vi "writeReadReg.vi"(6 "Bytes To Read":u8, 7 "I2C Channel":u8, 8 "error in":errorcluster, 9 "Data":u8[](array[numeric])=[0], 10 "I2C Slave Address":u8, 11 "LINX Resource in":T1) -> (0 "error out":errorcluster, 2 "Bytes Read":u8[](array[numeric]), 3 "LINX Resource out":T1)   [LabVIEW 2017]
uses:
  <vilib>/MakerHub/LINX/Private/Type Defs/LINX Ref.ctl
  <vilib>/MakerHub/LINX/Private/Type Defs/Platform.ctl
  <vilib>/MakerHub/LINX/Private/Type Defs/Interface.ctl
  <vilib>/MakerHub/LINX/Private/Device/Type Defs/LINX Device Config.ctl
  <vilib>/MakerHub/LINX/Private/Device/Type Defs/TCP Config.ctl
  <vilib>/MakerHub/LINX/Private/Device/Type Defs/Channels.ctl
  <vilib>/myRIO/Instrument Drivers/Onboard IO/I2C/typedefs/I2C User Configuration.ctl
  <vilib>/myRIO/Instrument Drivers/Onboard IO/I2C/typedefs/I2C Transfer Rate.ctl
  <vilib>/myRIO/Instrument Drivers/Onboard IO/I2C/typedefs/I2C Reference.ctl
  <vilib>/myRIO/Common/Instrument Driver Framework/Utilities/typedefs/myRIO Generic Hardware Reference.ctl
  <vilib>/myRIO/Common/Instrument Driver Framework/Utilities/typedefs/Hardware Version Enum.ctl
  <vilib>/myRIO/Common/Instrument Driver Framework/Utilities/typedefs/myRIO v1.0 Reference.ctl
  <vilib>/myRIO/Common/Instrument Driver Framework/Utilities/typedefs/Generic FPGA Reference.ctl
  <vilib>/myRIO/Common/Instrument Driver Framework/myRIO v1.0/I2C/typedefs/I2C Channels Enum.ctl
  <vilib>/myRIO/Instrument Drivers/Onboard IO/I2C/typedefs/I2C Configuration.ctl
  <vilib>/userdefined/High Color/nirio_resource_hc.ctl
  <vilib>/myRIO/Common/Instrument Driver Framework/Utilities/vis/Is FPGA Ref Available.vi
  <vilib>/myRIO/Common/Instrument Driver Framework/myRIO v1.0/I2C/vis/myRIO v1.1 Open I2C.vi
  <vilib>/MakerHub/LINX/Private/Local IO/LinxI2cWrite.vi
  <vilib>/MakerHub/LINX/Public/Utilities/Check Channel.vi
  <vilib>/myRIO/Common/Instrument Driver Framework/Utilities/vis/Validate Channels.vi
  <vilib>/myRIO/Common/Instrument Driver Framework/myRIO v1.0/I2C/vis/myRIO v1.0 Reserve I2C.vi
  <vilib>/myRIO/Common/Instrument Driver Framework/myRIO v1.0/I2C/vis/myRIO v1.0 Build MUX Configuration I2C.vi
  <vilib>/myRIO/Common/Instrument Driver Framework/myRIO v1.0/Resource Manager/vis/myRIO v1.0 Reserve Channel List.vi
  <vilib>/myRIO/Common/Instrument Driver Framework/myRIO v1.0/Resource Manager/vis/myRIO v1.0 Create Configuration List.vi
  <vilib>/myRIO/Common/Instrument Driver Framework/myRIO v1.0/Resource Manager/vis/myRIO v1.0 Reserve Channel.vi
  <vilib>/myRIO/Common/Instrument Driver Framework/myRIO v1.0/Resource Manager/vis/myRIO v1.0 Unreserve Channel.vi
  <vilib>/myRIO/Common/Instrument Driver Framework/myRIO v1.0/Resource Manager/vis/myRIO v1.0 Build Mutex Name.vi
  <vilib>/MakerHub/LINX/Private/Utilties/Generate Error.vi
  <vilib>/Utility/VariantDataType/GetNumericInfo.vi
  <vilib>/Utility/error.llb/Error Cluster From Error Code.vi
  <vilib>/myRIO/Common/Instrument Driver Framework/myRIO v1.0/myRIO v1.1 Open.vi
  <vilib>/myRIO/Common/Instrument Driver Framework/Utilities/vis/IO Manager.vi
  <vilib>/myRIO/Common/Instrument Driver Framework/Utilities/vis/Configuration Manager.vi
  <vilib>/myRIO/Common/Instrument Driver Framework/myRIO v1.0/Resource Manager/vis/myRIO v1.0 Configure IO.vi
  <vilib>/myRIO/Common/Instrument Driver Framework/myRIO v1.0/myRIO v1.0 Close.vi
  <vilib>/myRIO/Common/Instrument Driver Framework/myRIO v1.0/I2C/vis/myRIO v1.0 Configure I2C.vi
  <vilib>/myRIO/Common/Instrument Driver Framework/myRIO v1.0/I2C/vis/myRIO v1.0 Write I2C.vi
  <vilib>/myRIO/Common/Instrument Driver Framework/myRIO v1.0/I2C/vis/myRIO v1.0 Read I2C.vi
  <vilib>/myRIO/Express VI/Onboard IO/I2C/I2C Express VI.xnode
  <vilib>/myRIO/Instrument Drivers/Onboard IO/I2C/vis/myRIO I2C Open.xnode
  <vilib>/myRIO/Instrument Drivers/Onboard IO/I2C/I2C.lvlib
  <vilib>/MakerHub/LINX/LMH-LINX.lvlib
  <vilib>/MakerHub/LINX/Private/Device/Device.lvlib
panel:
  in  "I2C Impl.":enum16{"LINX", "myRIO Express", "myRIO subVIs"}(ring)=enum."myRIO subVIs"
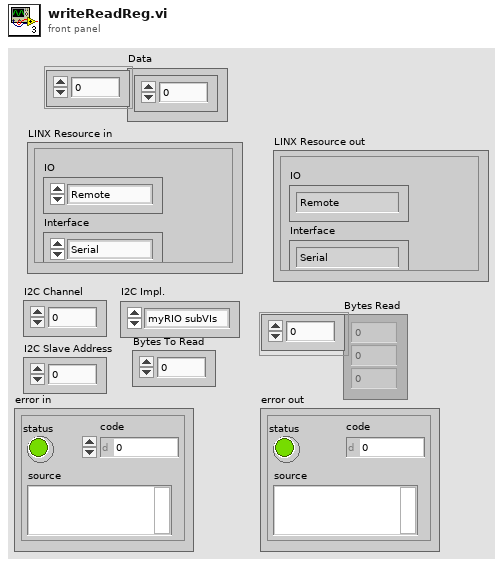
[diagram p1: front panel]
types:
  T1 = typedef "LMH-LINX.lvlib/LINX Ref.ctl" = cluster{"IO":T2, "Interface":T3, "LINX Device Config":T4}
  T2 = typedef "LMH-LINX.lvlib/Platform.ctl" = enum16{"Remote", "Local"}
  T3 = typedef "LMH-LINX.lvlib/Interface.ctl" = enum16{"Serial", "TCP"}
  T4 = typedef "LMH-LINX.lvlib/Device.lvlib/LINX Device Config.ctl" = cluster{"Interface":T3, "COM Port":refnum<visa-resource-name>, "TCP Configuration":T5, "Device Family":u8, "Device ID":u8, "Device Name":string, "TCP Ref":refnum<k5>, "Channels":T6}
  T5 = typedef "LMH-LINX.lvlib/Device.lvlib/TCP Config.ctl" = cluster{"IP Address":string, "Port":u16}
  T6 = typedef "LMH-LINX.lvlib/Channels.ctl" = cluster{"DI":u8[], "DO":u8[], "AI":u8[], "AO":u8[], "PWM":u8[], "QE":u8[], "UART":u8[], "I2C 2":u8[], "SPI":u8[], "CAN":u8[], "Servo":u8[], "AI Ref (V)":dbl, "AI Resolution (Bits)":u8, "AO Ref (V)":dbl, "AO Resolution (Bits)":u8}
  T7 = typedef "I2C.lvlib/I2C Reference.ctl" = cluster{"myRIO Reference":T8, "I2C Channels Enum":T12, "I2C Configuration":T13}
  T8 = typedef "myRIO Generic Hardware Reference.ctl" = cluster{"myRIO Model":T9, "myRIO Hardware Reference":T10}
  T9 = typedef "Hardware Version Enum.ctl" = enum16{"Unknown", "myRIO-1900", "myRIO-1950", "roboRIO", "NI ELVIS RIO CM"}
  T10 = typedef "myRIO v1.0 Reference.ctl" = cluster{"Generic FPGA Reference":T11, "Allow multiple opens":bool}
  T11 = typedef "Generic FPGA Reference.ctl" = refnum<k20>
  T12 = typedef "I2C Channels Enum.ctl" = enum16{"Not Connected", "A/I2C", "B/I2C", "I2C/I2C"}
  T13 = typedef "I2C.lvlib/I2C Configuration.ctl" = cluster{"I2C Transfer Rate":T14}
  T14 = typedef "I2C.lvlib/I2C Transfer Rate.ctl" = enum16{"Standard mode (100 kbps)", "Fast mode (400 kbps)"}
  T15 = typedef "I2C.lvlib/I2C User Configuration.ctl" = cluster{"I2C Transfer Rate":T14}
  T16 = typedef "nirio_resource_hc.ctl" = tag
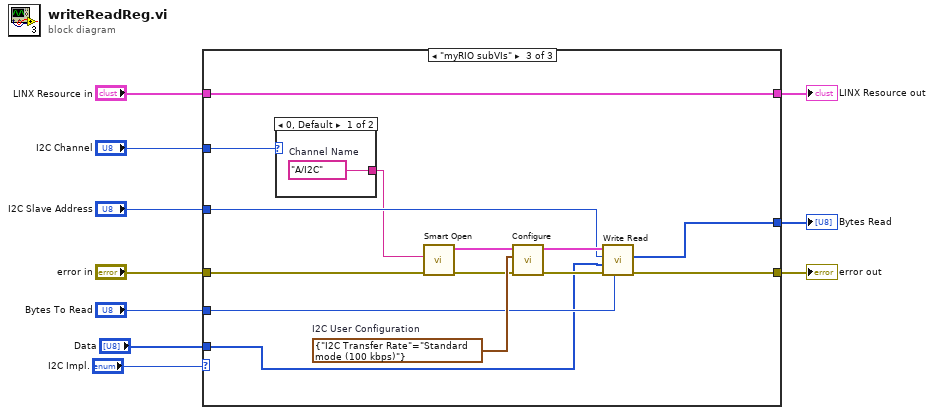
[diagram p0: block diagram]
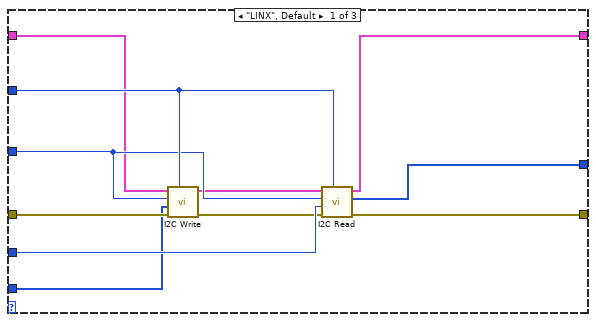
[diagram p2: hidden frame]
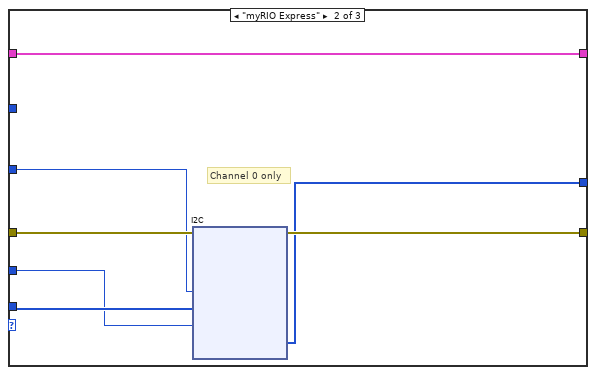
[diagram p3: hidden frame]
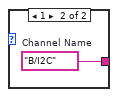
[diagram p4: hidden frame]
diagram:
  n1 = case shown="\"myRIO subVIs\"" "I2C Impl." {
    tunnel: [w20 w25 w81] -> w10
    tunnel: "error in" -> [w16 w27 w76]
    tunnel: [w21 w26 w69] -> w8
    tunnel: "I2C Slave Address" -> [w13 w24 w75]
    tunnel: "Bytes To Read" -> [w18 w22 w74]
    tunnel: "I2C Channel" -> [w14 _ w73]
    tunnel: "LINX Resource in" -> [w12 w28 w72]
    tunnel: [w19 w28 w72] -> w2
    tunnel: "Data" -> [w15 w23 w71]
    frame "LINX", Default {
      n2 = call <vilib>:"I2C Write.vi"("I2C Channel"=w14, "Error In"=w16, "Data"=w15, "I2C Slave Address (0)"=w13, "LINX Resource"=w12) -> ("Error Out"=w17:errorcluster, "LINX Resource"=w11:T1)  [unwired: 5 in]
      n3 = call <vilib>:"I2C Read.vi"("I2C Channel"=w14, "Error In"=w17, "Bytes To Read"=w18, "I2C Slave Address (0)"=w13, "LINX Resource"=w11) -> ("Error Out"=w21:errorcluster, "Data"=w20:u8[], "LINX Resource"=w19:T1)  [unwired: 4 in]
    }
    frame "myRIO Express" {
      # "Channel 0 only"
      n4 = xnode "I2C"("Slave Address (7-bit)"=w24, "Bytes to Write"=w23, "Byte Count"=w22, "error in (no error)"=w27) -> ("Bytes Read"=w25:u8[], "error out"=w26:errorcluster)
    }
    frame "myRIO subVIs" {
      w82 = T15 {"I2C Transfer Rate"=enum."Standard mode (100 kbps)"}  # I2C User Configuration
      n5 = case shown="0, Default" w73 {
        tunnel: [w83 w84] -> w70
        frame 0, Default {
          w83 = tag "A/I2C"  # Channel Name
        }
        frame 1 {
          w84 = tag "B/I2C"  # Channel Name
        }
      }
      n6 = call <vilib>:"Smart Open.vi"("error in (no error)"=w76, "Channel Name"=w70) -> ("error out"=w79:errorcluster, "I2C Ref Out"=w80:T7)  [unwired: 8 in]
      n7 = call <vilib>:"Configure.vi"("error in (no error)"=w79, "I2C User Configuration"=w82, "I2C Ref In"=w80) -> ("error out"=w77:errorcluster, "I2C Ref Out"=w78:T7)  [unwired: 7 in]
      n8 = call <vilib>:"Write Read.vi"("Byte Count"=w74, "error in (no error)"=w77, "Bytes to Write"=w71, "Slave Address (7-bit)"=w75, "I2C Ref In"=w78) -> ("error out"=w69:errorcluster, "Bytes Read"=w81:u8[])  [unwired: 3 in, 1 out]
    }
  }
  "error out" <- w8
  "LINX Resource out" <- w2
  "Bytes Read" <- w10
